vi "EXA_registerCallback_Summary.vi"(8 "error in (no error)":errorcluster, 10 "skipOld":bool, 11 "handle":i32) -> (0 "error out":errorcluster, 3 "function return":i32)   [LabVIEW 2016, in "SALLV_EXA.lvlib"]
doc: "int EXA_shm_registerCallback_SummaryLV(int handle, bool skipOld);"
uses:
  SALLV_EXA.lvlib
  SALLV_EXA.so
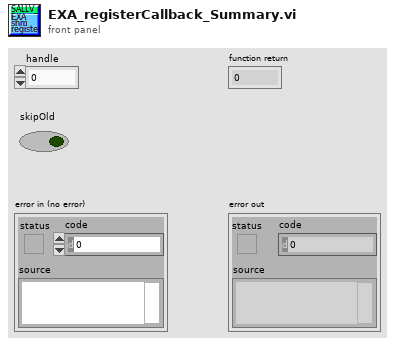
[diagram p1: front panel]
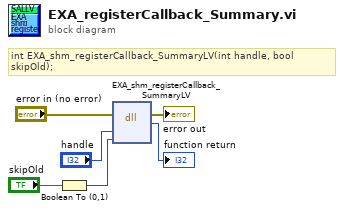
[diagram p0: block diagram]
diagram:
  # "int EXA_shm_registerCallback_SummaryLV(int handle, bool skipOld);"
  n1 = Boolean To (0,1)(Boolean="skipOld") -> (0, 1=w3:i16)
  n2 = dll-call lib="home/hsundar/TCS/EXA/SALLV_EXA/SALLV_EXA.*" fn="EXA_shm_registerCallback_SummaryLV"(error in="error in (no error)", "handle"="handle", "skipOld"=w3) -> (error out=→"error out":errorcluster, →"function return":i32)  [unwired: 4 in, 1 out]
